vi "SIM_FrameProperties.vi"() -> (0 "data":dbl[][](array[numeric]), 2 "Size (m)":cluster{"Width":sgl, "Height":sgl} {"Height" format="%.2p"; "Width" format="%.2p"}, 3 "Origin (m)":cluster{"Xc":sgl, "Yc":sgl} {"Yc" format="%.2p"; "Xc" format="%.2p"})   [LabVIEW 2019]
uses:
  <vilib>/Utility/file.llb/Read Delimited Spreadsheet (DBL).vi
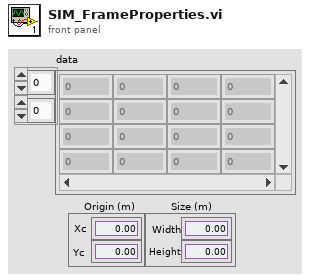
[diagram p1: front panel]
types:
  T1 = cluster{"[0]":dbl, "[1]":dbl, "[2]":dbl, "[3]":dbl, "[4]":dbl, "[5]":dbl, "[6]":dbl, "[7]":dbl, "[8]":dbl}
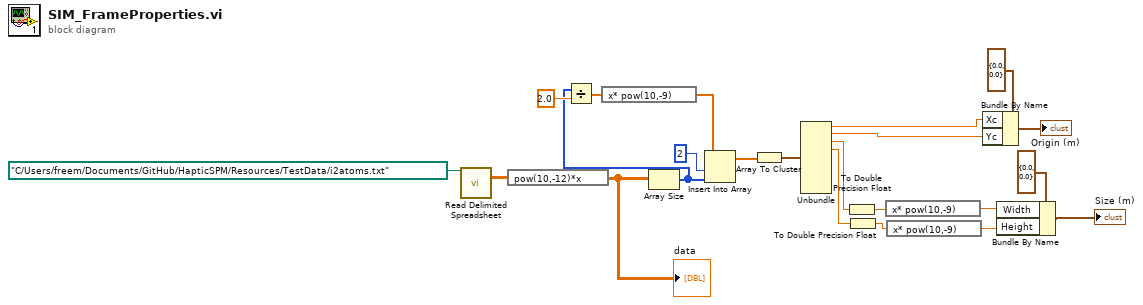
[diagram p0: block diagram]
diagram:
  n1 = call-poly <vilib>:"Read Delimited Spreadsheet.vi"("file path (dialog if empty)"=path "C:/Users/freem/Documents/GitHub/HapticSPM/Resources/TestData/i2atoms.txt") -> ("all rows"=w19:dbl[][])  [unwired: 9 in, 5 out]
  n2 = expression code="pow(10,-12)*x"(w19) -> (w18:dbl[][])
  "data" <- w18
  n3 = Array Size(array=w18) -> (size(s)=w4:i32[])
  n4 = Divide(x=w4, y=2.0) -> (x/y=w2:dbl[])
  n5 = expression code="x* pow(10,-9)"(w2) -> (w1:dbl[])
  n6 = Insert Into Array(array=w1, index=2, new element=w4) -> (w3:dbl[])
  n7 = Array To Cluster(array=w3) -> (cluster=w20:T1)
  n8 = Unbundle(w20) -> ("[0]"=w16:dbl, "[1]"=w15:dbl, "[2]"=w9:dbl, "[3]"=w8:dbl)  [unwired: 5 out]
  n9 = To Double Precision Float(number=w9) -> (double precision float=w7:dbl)
  n10 = To Double Precision Float(number=w8) -> (double precision float=w6:dbl)
  n11 = expression code="x* pow(10,-9)"(w7) -> (w11:dbl)
  n12 = expression code="x* pow(10,-9)"(w6) -> (w10:dbl)
  n13 = Bundle By Name(cluster=cluster{"Xc":sgl, "Yc":sgl} {"Xc"=0.0, "Yc"=0.0} ("Origin (m)"), "Xc"=w16, "Yc"=w15) -> (→"Origin (m)":cluster{"Xc":sgl, "Yc":sgl})
  n14 = Bundle By Name(cluster=cluster{"Width":sgl, "Height":sgl} {"Width"=0.0, "Height"=0.0} ("Size (m)"), "Width"=w11, "Height"=w10) -> (→"Size (m)":cluster{"Width":sgl, "Height":sgl})
